vi "DRAW_Track_overlays_(offline).vi"(0 "Image size":cluster{"x":i32, "y":i32}={"x"=480, "y"=480}, 5 "Full track array":T1(array[cluster]), 7 "Speed array":dbl[](array[numeric]), 11 "Error In":errorcluster) -> (4 "Time-coded overlay pixmap":u32[][](array[numeric]) format="%x", 6 "Speed-coded overlay pixmap":u32[][](array[numeric]) format="%x", 8 "Plain track overlay pixmap":u32[][](array[numeric]) format="%x", 15 "Error Out":errorcluster)   [LabVIEW 2018, in "Tracker.lvlib"]
uses:
  Tracker.lvlib
panel:
  in  "Lower bound":cluster{"x":i32, "y":i32}
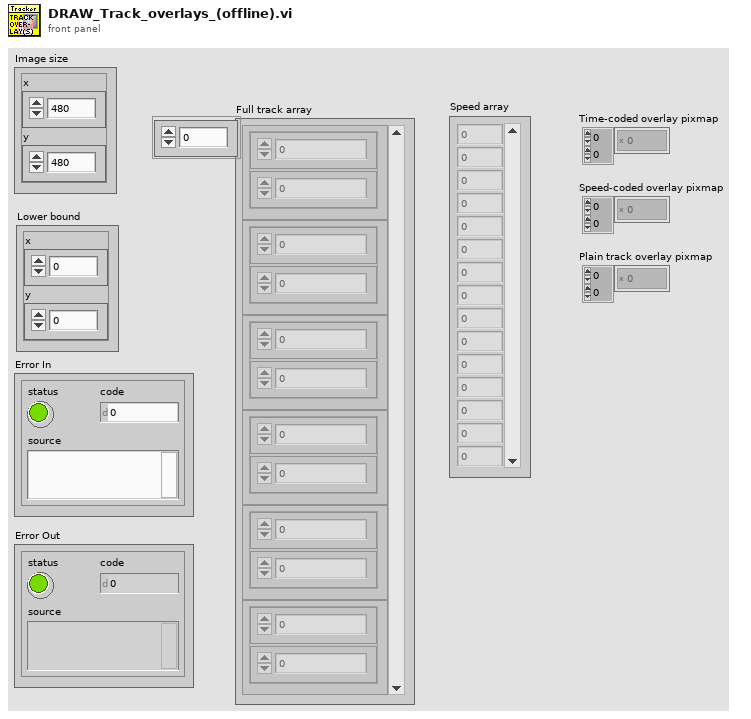
[diagram p1: front panel]
types:
  T1 = cluster{"Numeric Control":dbl, "Numeric Control":dbl}[]
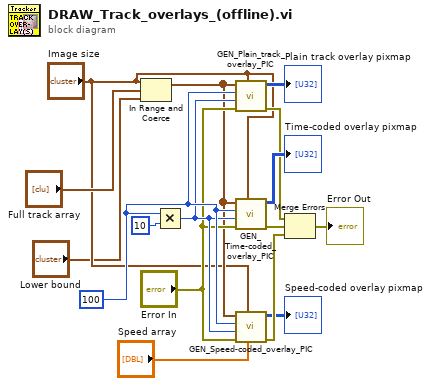
[diagram p0: block diagram]
diagram:
  w8 = 100 ("Multiline grouping")
  n1 = In Range and Coerce(upper limit="Image size", x="Full track array", lower limit="Lower bound") -> (coerced(x)=w3:T1)  [unwired: 1 out]
  n2 = Multiply(x=w8, y=10) -> (x*y=w7:i32)
  n3 = call "GEN_Plain_track_overlay_PIC.vi"("Image size"="Image size", "Error In"="Error In", "Samples full merge, every N"=w7, "Multiline grouping, samples"=w8, "Full track array"=w3) -> ("Error Out"=w5:errorcluster, "Plain track overlay pixmap"=→"Plain track overlay pixmap":u32[][])  [unwired: 5 in]
  n4 = call "GEN_Time-coded_overlay_PIC.vi"("Image size"="Image size", "Error In"="Error In", "Samples full merge, every N"=w7, "Multiline grouping, samples"=w8, "Full track array"=w3) -> ("Error Out"=w13:errorcluster, "Time-coded overlay pixmap"=→"Time-coded overlay pixmap":u32[][])  [unwired: 5 in]
  n5 = call "GEN_Speed-coded_overlay_PIC.vi"("Speed array in"="Speed array", "Image size"="Image size", "Error In"="Error In", "Samples full merge, every N"=w7, "Multiline grouping, samples"=w8, "Full track array"=w3) -> ("Error Out"=w12:errorcluster, "Speed-coded overlay pixmap"=→"Speed-coded overlay pixmap":u32[][])  [unwired: 4 in]
  n6 = Merge Errors(w5, w13, w12) -> (→"Error Out":errorcluster)
